vi "Begin Bin.vi"   [LabVIEW 2018, in "Toolkit.lvlib" / "Reader.lvclass"]
doc: "Starts reading, but does not decode, a binary blob from the MessagePack data. Use the Read Bytes VI to obtain the binary blob."
uses:
  Reader.lvclass
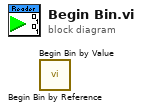
[diagram p0: block diagram]
diagram:
  n1 = call "Begin Bin by Reference.vi"() -> ()  [unwired: 9 in, 3 out]
  n2 = call "Begin Bin by Value.vi"() -> ()  [unwired: 9 in, 3 out]
